vi "登陆主界面 .vi"() -> ()   [LabVIEW 2015]
panel:
  in  "VI路径 2":path=path "D:/搜狗高速下载/LabVIEW/labview资料/登录界面/登录界面/密码修改.vi"
  out "滑动杆":u8(slide) scale=0.0..100.0
  in  "VI路径":path=path "D:/搜狗高速下载/LabVIEW/labview资料/登录界面/登录界面/要进入系统的界面.vi"
  in  "原密码所在位置":path=path "D:/搜狗高速下载/LabVIEW/labview资料/登录界面/登录界面/user.txt"
  in  "修改密码":bool
  in  "退出":bool
  in  "登陆":bool
  in  "密码：":string
  in  "账户：":string
  # "登录系统"
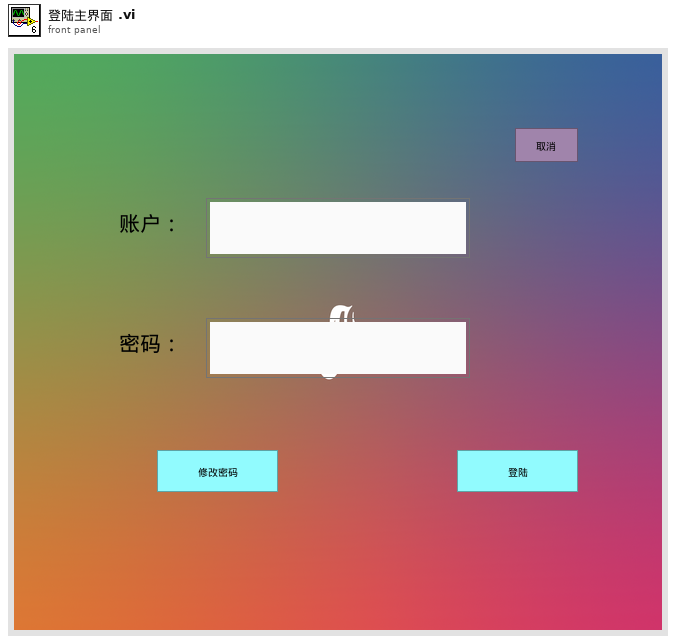
[diagram p1: front panel]
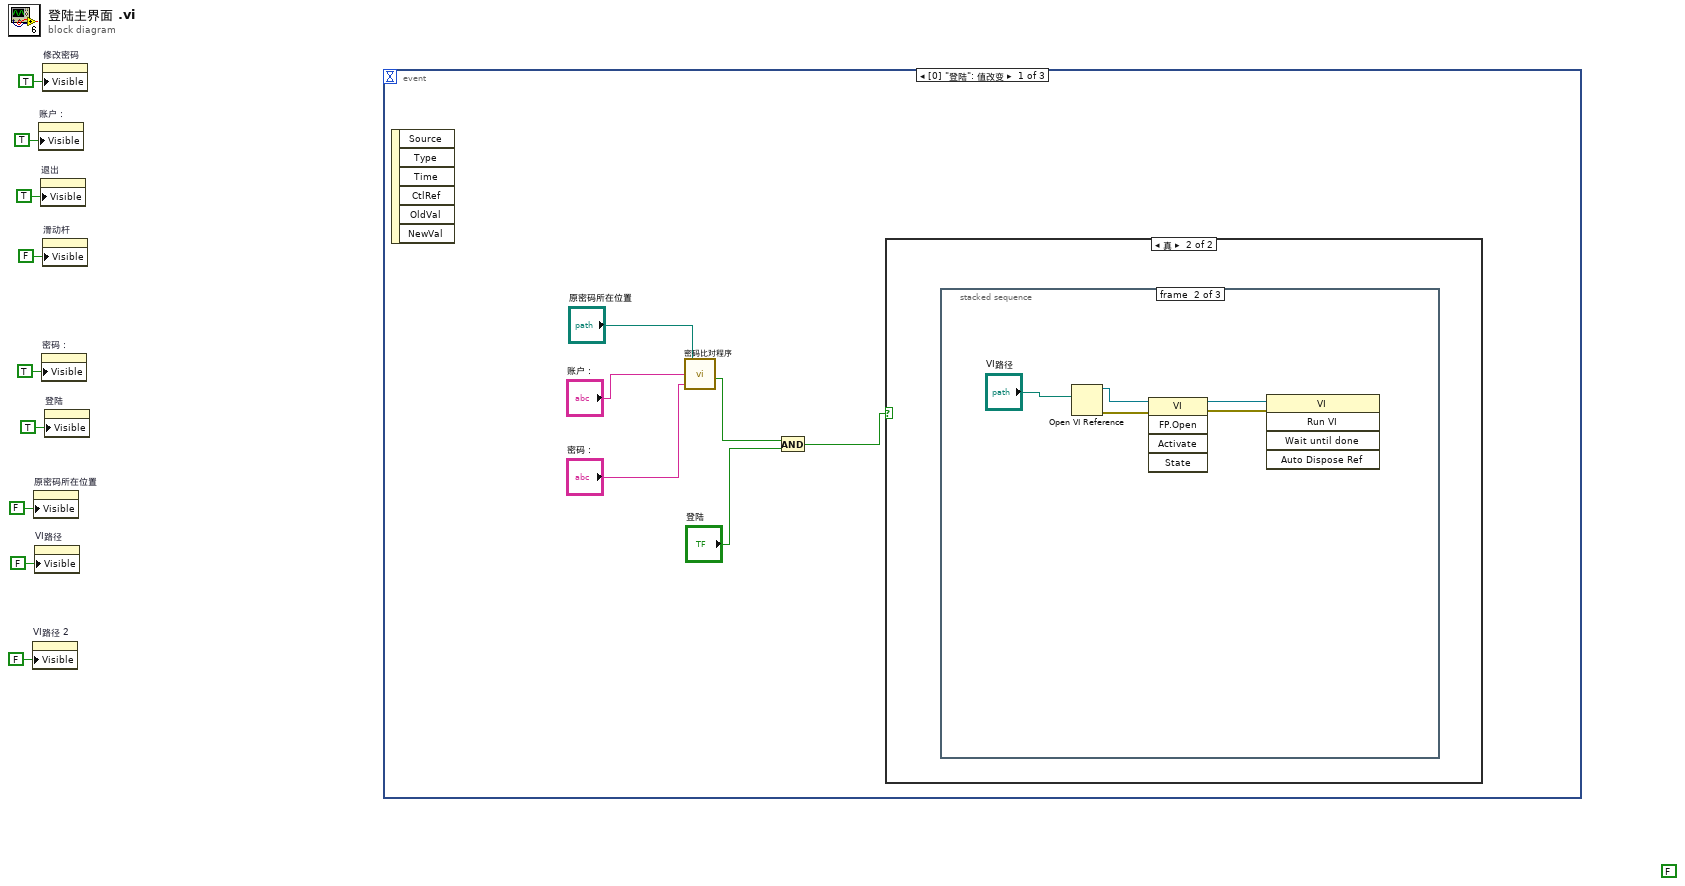
[diagram p0: block diagram]
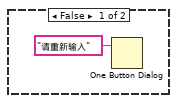
[diagram p2: hidden frame]
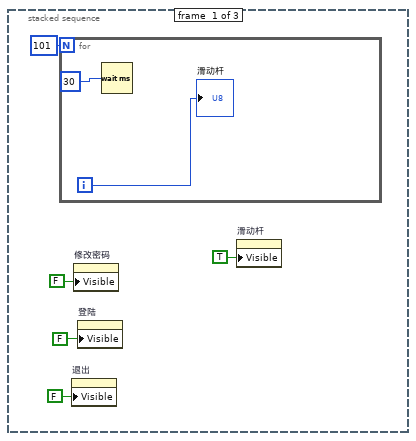
[diagram p3: hidden frame]
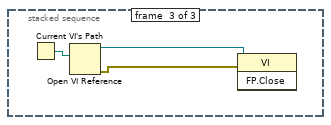
[diagram p4: hidden frame]
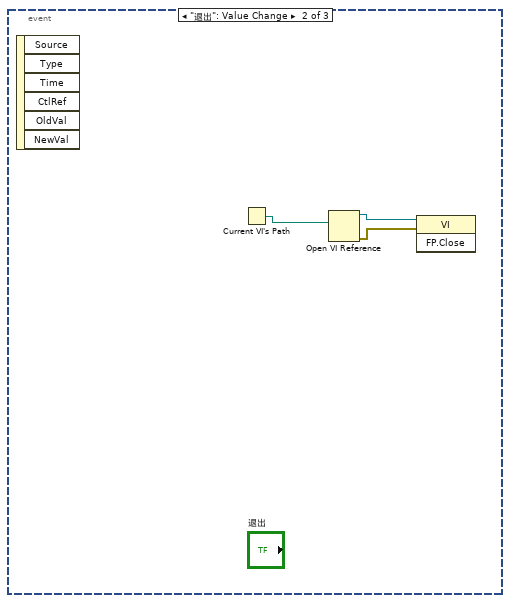
[diagram p5: hidden frame]
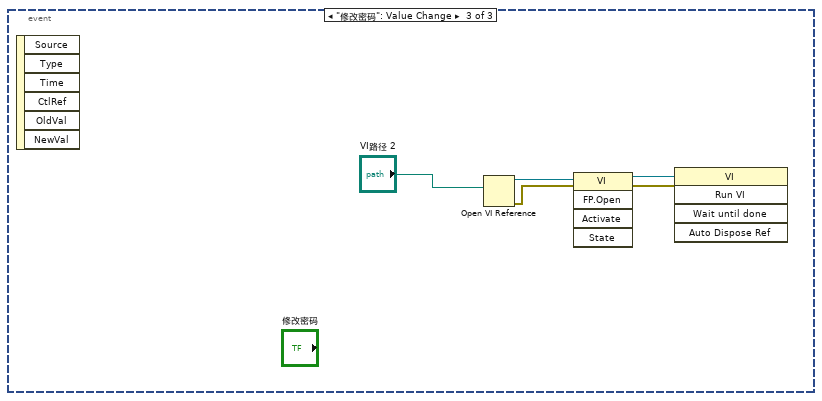
[diagram p6: hidden frame]
diagram:
  (unwired) FALSE
  n1 = property on="VI路径 2" class="Path"("Visible"=FALSE ("可见")) -> ()  [unwired: 2 in, 2 out]
  n2 = property on="原密码所在位置" class="Path"("Visible"=FALSE ("可见")) -> ()  [unwired: 2 in, 2 out]
  n3 = property on="VI路径" class="Path"("Visible"=FALSE ("可见")) -> ()  [unwired: 2 in, 2 out]
  n4 = property on="账户：" class="Str"("Visible"=TRUE ("可见")) -> ()  [unwired: 2 in, 2 out]
  n5 = property on="退出" class="Bool"("Visible"=TRUE ("可见")) -> ()  [unwired: 2 in, 2 out]
  n6 = property on="密码：" class="Str"("Visible"=TRUE ("可见")) -> ()  [unwired: 2 in, 2 out]
  n7 = property on="修改密码" class="Bool"("Visible"=TRUE ("可见")) -> ()  [unwired: 2 in, 2 out]
  n8 = property on="滑动杆" class="Slide (严格)"("Visible"=FALSE ("可见")) -> ()  [unwired: 2 in, 2 out]
  n9 = property on="登陆" class="Bool"("Visible"=TRUE ("可见")) -> ()  [unwired: 2 in, 2 out]
  n10 = event shown="[0] \"登陆\": 值改变" {
    selector: _ -> [_ _ _]
    dyn-events: _ -> [_ _ _]
    timeout: _ -> [_ _ _]
    event "登陆": Value Change {
      n11 = event-data() -> ()  [unwired: 1 in, 6 out]
      n12 = call "密码比对程序.vi"("密码"="密码：", "账户"="账户：", "原密码所在位置"="原密码所在位置") -> ("x = y?"=w11:bool)  [unwired: 5 in]
      n13 = And(x=w11, y="登陆") -> (x .and. y?=w10:bool)
      n14 = case shown="真" w10 {
        frame False {
          n15 = One Button Dialog(message="请重新输入" ("消息")) -> ()  [unwired: 1 in, 1 out]
        }
        frame True {
          n16 = stacked-sequence {
            frame #0 {
              n17 = for {
                N: 101 -> [_]
                i -> [w23]
                n18 = Wait (ms)(milliseconds to wait=u32 30 ("等待时间（毫秒）")) -> ()  [unwired: 1 out]
                "滑动杆" <- w23
              }
              n19 = property on="退出" class="Bool"("Visible"=FALSE ("可见")) -> ()  [unwired: 2 in, 2 out]
              n20 = property on="修改密码" class="Bool"("Visible"=FALSE ("可见")) -> ()  [unwired: 2 in, 2 out]
              n21 = property on="登陆" class="Bool"("Visible"=FALSE ("可见")) -> ()  [unwired: 2 in, 2 out]
              n22 = property on="滑动杆" class="Slide (严格)"("Visible"=TRUE ("可见")) -> ()  [unwired: 2 in, 2 out]
            }
            frame #1 {
              n23 = Open VI Reference(vi path="VI路径") -> (vi reference=w28:refnum<vi>, error out=w27:errorcluster)  [unwired: 5 in]
              n24 = invoke class="VI" method="FP.Open"(reference=w28, error in=w27) -> (reference out=w25:refnum<vi>, error out=w24:errorcluster)  [unwired: 3 in, 3 out]
              n25 = invoke class="VI" method="Run VI"(reference=w25, error in=w24) -> ()  [unwired: 3 in, 5 out]
            }
            frame #2 {
              n26 = Current VI's Path() -> (path=w29:path)
              n27 = Open VI Reference(vi path=w29) -> (vi reference=w30:refnum<vi>, error out=w31:errorcluster)  [unwired: 5 in]
              n28 = invoke class="VI" method="FP.Close"(reference=w30, error in=w31) -> ()  [unwired: 1 in, 3 out]
            }
          }
        }
      }
    }
    event "退出": Value Change {
      n29 = event-data() -> ()  [unwired: 1 in, 6 out]
      n30 = Current VI's Path() -> (path=w32:path)
      n31 = Open VI Reference(vi path=w32) -> (vi reference=w34:refnum<vi>, error out=w33:errorcluster)  [unwired: 5 in]
      n32 = invoke class="VI" method="FP.Close"(reference=w34, error in=w33) -> ()  [unwired: 1 in, 3 out]
    }
    event "修改密码": Value Change {
      n33 = event-data() -> ()  [unwired: 1 in, 6 out]
      n34 = Open VI Reference(vi path="VI路径 2") -> (vi reference=w38:refnum<vi>, error out=w37:errorcluster)  [unwired: 5 in]
      n35 = invoke class="VI" method="FP.Open"(reference=w38, error in=w37) -> (reference out=w36:refnum<vi>, error out=w35:errorcluster)  [unwired: 3 in, 3 out]
      n36 = invoke class="VI" method="Run VI"(reference=w36, error in=w35) -> ()  [unwired: 3 in, 5 out]
    }
  }
